vi "My_RIGOL.vi"() -> ()   [LabVIEW 2012]
uses:
  RIGOL DG4000 Series.lvlib
panel:
  out "String 4":string
  out "String 3":string
  out "String 2":string
  out "String":string
  in  "Количество точек":dbl
  in  "Время между импульсами, с":dbl
  in  "Ширина импульса, с":dbl=1000.0
  out "Выход на канал 2":string
  out "Выход на канал 1":string
  in  "Amplitude Unit (0: Vpp) 2":i32(ring) items=["Vpp", "Vrms", "dBm"]
  in  "Amplitude (5 Vpp) 2":dbl=5.0
  in  "Amplitude Unit (0: Vpp)":i32(ring) items=["Vpp", "Vrms", "dBm"]
  in  "Amplitude (5 Vpp)":dbl=5.0
  in  "Частота (1000 Hz)":dbl=1000.0
  in  "VISA resource name":refnum<visa-resource-name>
  # "Chanel 2"
  # "Chanel 1"
  # "ДИОД"
  # "ДЕТЕКТОР"
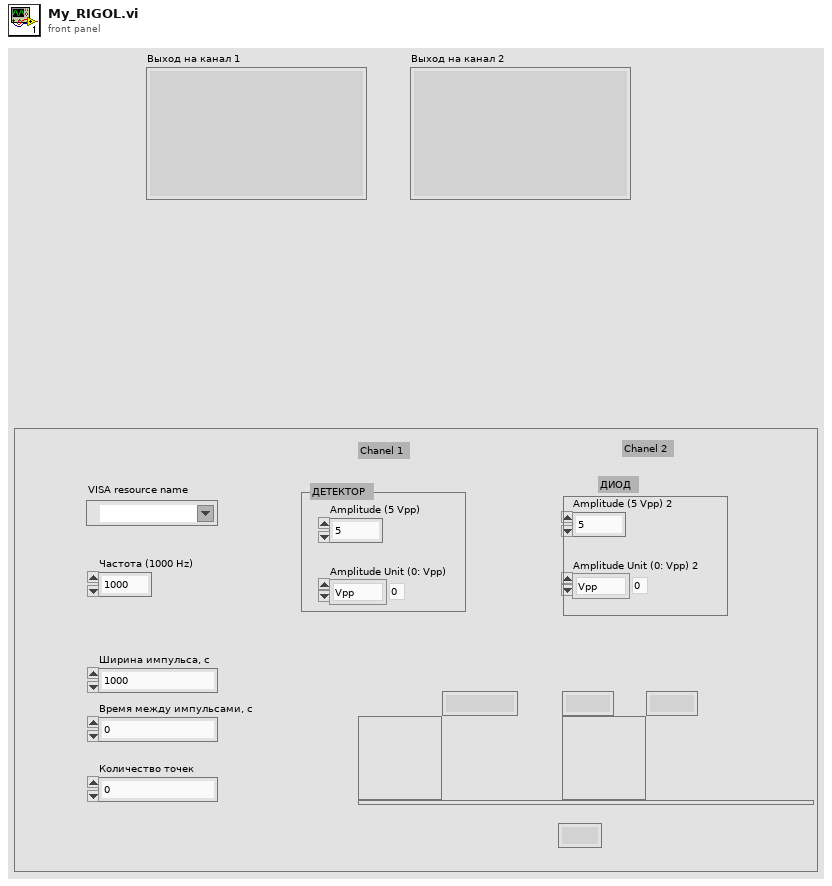
[diagram p1: front panel]
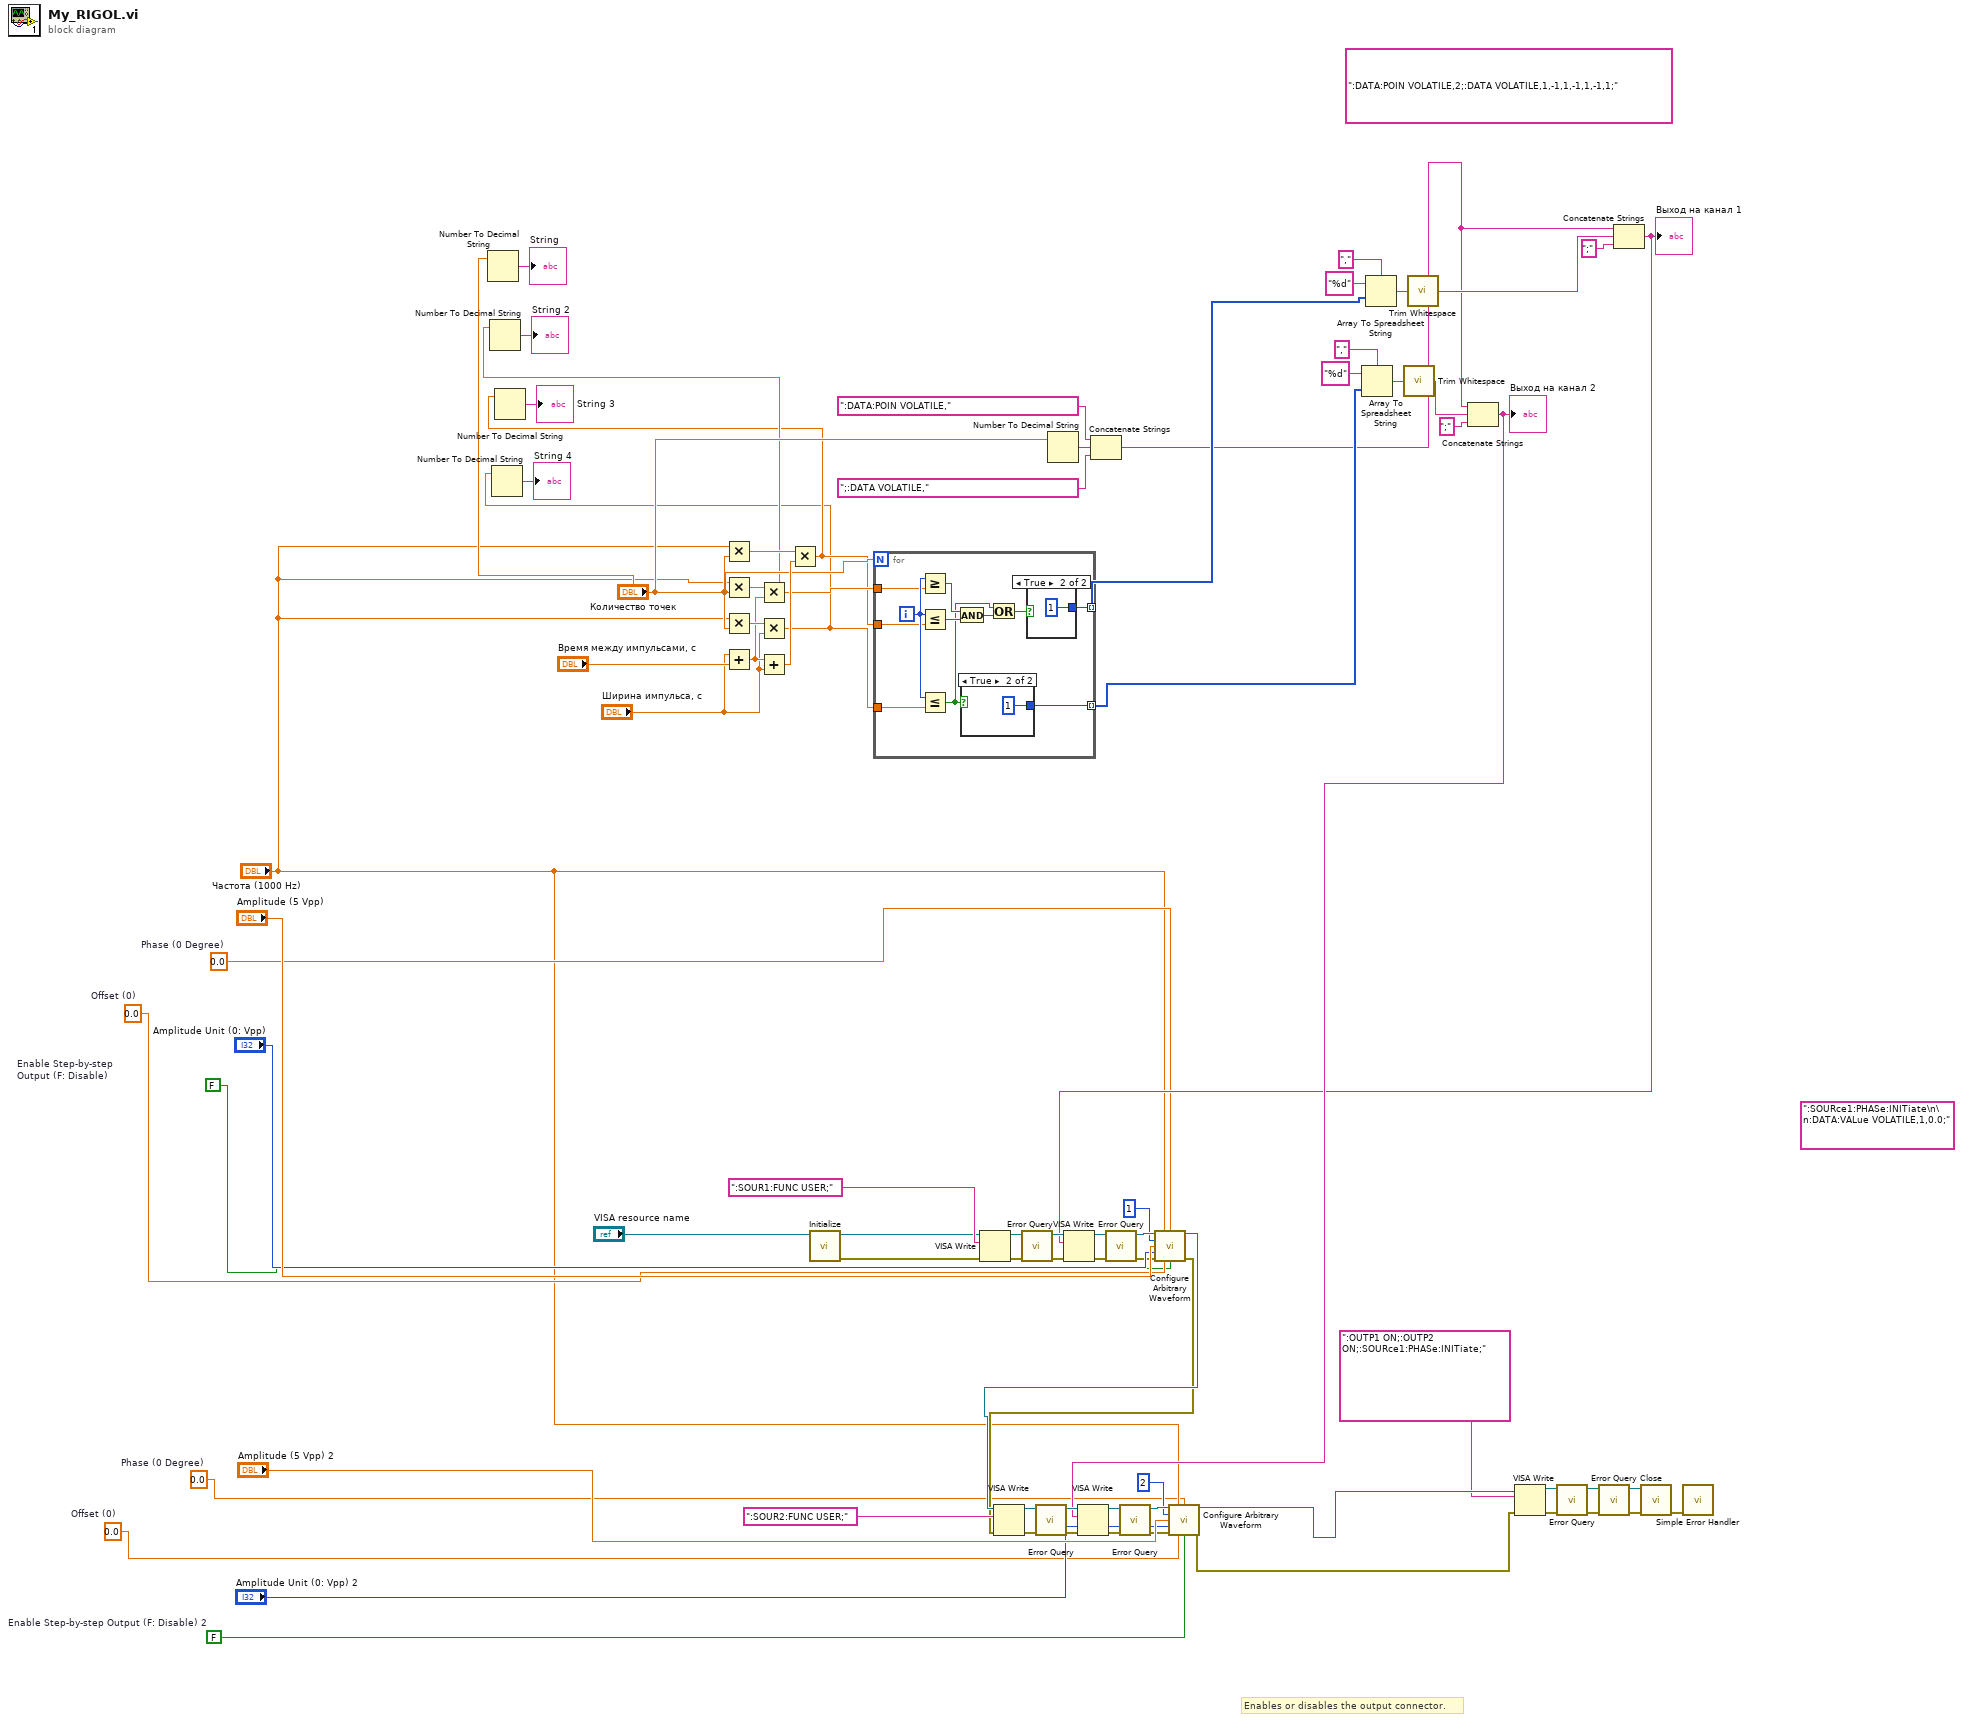
[diagram p0: block diagram]
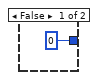
[diagram p2: hidden frame]
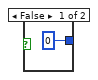
[diagram p3: hidden frame]
diagram:
  w1 = FALSE  # Enable Step-by-step Output (F: Disable) 2
  w2 = FALSE  # Enable Step-by-step Output (F: Disable)
  w3 = 0.0  # Offset (0)
  w4 = 0.0  # Phase (0 Degree)
  w6 = 0.0  # Offset (0)
  w7 = 0.0  # Phase (0 Degree)
  (unwired) ":SOURce1:PHASe:INITiate\n\n:DATA:VALue VOLATILE,1,0.0;"
  (unwired) ":DATA:POIN VOLATILE,2;:DATA VOLATILE,1,-1,1,-1,1,-1,1;"
  # "Enables or disables the output connector."
  n1 = Number To Decimal String(number="Количество точек") -> (decimal integer string=→"String":string)  [unwired: 1 in]
  n2 = Multiply(x="Частота (1000 Hz)", y="Количество точек") -> (x*y=w17:dbl)
  n3 = Multiply(x="Частота (1000 Hz)", y="Количество точек") -> (x*y=w21:dbl)
  n4 = Multiply(x="Частота (1000 Hz)", y="Количество точек") -> (x*y=w22:dbl)
  n5 = Add(x="Ширина импульса, с", y="Время между импульсами, с") -> (x+y=w19:dbl)
  n6 = Multiply(x=w21, y=w19) -> (x*y=w10:dbl)
  n7 = Number To Decimal String(number=w10) -> (decimal integer string=→"String 2":string)  [unwired: 1 in]
  n8 = Multiply(x=w22, y="Ширина импульса, с") -> (x*y=w8:dbl)
  n9 = Number To Decimal String(number=w8) -> (decimal integer string=→"String 4":string)  [unwired: 1 in]
  n10 = Add(x=w19, y="Ширина импульса, с") -> (x+y=w16:dbl)
  n11 = Multiply(x=w17, y=w16) -> (x*y=w9:dbl)
  n12 = Number To Decimal String(number=w9) -> (decimal integer string=→"String 3":string)  [unwired: 1 in]
  n13 = call "Initialize.vi"("VISA resource name"="VISA resource name") -> ("error out"=w50:errorcluster, "VISA resource name out"=w51:refnum<visa-resource-name>)  [unwired: 4 in, 5 out]
  n14 = for {
    N: "Количество точек" -> [_]
    tunnel: [w90] -> w38 mode=indexing
    tunnel: w8 -> [w89]
    tunnel: w10 -> [w83]
    tunnel: w9 -> [w82]
    tunnel: [w80] -> w31 mode=indexing
    i -> [w84]
    n15 = Greater Or Equal?(x=w84, y=w83) -> (x >= y?=w86:bool)
    n16 = Less Or Equal?(x=w84, y=w82) -> (x <= y?=w85:bool)
    n17 = Less Or Equal?(x=w84, y=w89) -> (x <= y?=w81:bool)
    n18 = And(x=w86, y=w85) -> (x .and. y?=w88:bool)
    n19 = case shown="True" w81 {
      tunnel: [0 1] -> w80
      frame False {
      }
      frame True {
      }
    }
    n20 = Or(x=w81, y=w88) -> (x .or. y?=w87:bool)
    n21 = case shown="True" w87 {
      tunnel: [0 1] -> w90
      frame False {
      }
      frame True {
      }
    }
  }
  n22 = VISA Write(VISA resource name=w51, write buffer=":SOUR1:FUNC USER;", error in (no error)=w50) -> (VISA resource name out=w75:refnum<visa-resource-name>, error out=w73:errorcluster)  [unwired: 1 out]
  n23 = call "Error Query.vi"("error in (no error)"=w73, "VISA resource name"=w75) -> ("error out"=w67:errorcluster, "VISA resource name out"=w70:refnum<visa-resource-name>)  [unwired: 8 out]
  n24 = Number To Decimal String(number="Количество точек") -> (decimal integer string=w28:string)  [unwired: 1 in]
  n25 = Concatenate Strings(":DATA:POIN VOLATILE,", w28, ";:DATA VOLATILE,") -> (w25:string)
  n26 = Array To Spreadsheet String(delimiter (Tab)=",", array=w31, 3:"%d") -> (spreadsheet string=w33:string)
  n27 = Array To Spreadsheet String(delimiter (Tab)=",", array=w38, 3:"%d") -> (spreadsheet string=w39:string)
  n28 = call <vilib>:"Trim Whitespace.vi"("string"=w33) -> ("trimmed string"=w32:string)  [unwired: 1 in]
  n29 = call <vilib>:"Trim Whitespace.vi"("string"=w39) -> ("trimmed string"=w37:string)  [unwired: 1 in]
  n30 = Concatenate Strings(w25, w32, ";" ("delimiter (Tab)")) -> (w30:string)
  "Выход на канал 2" <- w30
  n31 = Concatenate Strings(w25, w37, ";" ("delimiter (Tab)")) -> (w29:string)
  "Выход на канал 1" <- w29
  n32 = VISA Write(VISA resource name=w70, write buffer=w29, error in (no error)=w67) -> (VISA resource name out=w69:refnum<visa-resource-name>, error out=w66:errorcluster)  [unwired: 1 out]
  n33 = call "Error Query.vi"("error in (no error)"=w66, "VISA resource name"=w69) -> ("error out"=w65:errorcluster, "VISA resource name out"=w68:refnum<visa-resource-name>)  [unwired: 8 out]
  n34 = call "Configure Arbitrary Waveform.vi"("VISA resource name"=w68, "Frequency (1000 Hz)"="Частота (1000 Hz)", "Phase (0 Degree)"=w7, "Output Channel (1: Channel 1)"=1, "Amplitude (5 Vpp)"="Amplitude (5 Vpp)", "Amplitude Unit (0: Vpp)"="Amplitude Unit (0: Vpp)", "error in (no error)"=w65, "Offset (0)"=w6, "Enable Step-by-step Output (F: Disable)"=w2) -> ("VISA resource name out"=w53:refnum<visa-resource-name>, "error out"=w52:errorcluster)  [unwired: 5 in]
  n35 = VISA Write(VISA resource name=w53, write buffer=":SOUR2:FUNC USER;", error in (no error)=w52) -> (VISA resource name out=w64:refnum<visa-resource-name>, error out=w62:errorcluster)  [unwired: 1 out]
  n36 = call "Error Query.vi"("error in (no error)"=w62, "VISA resource name"=w64) -> ("error out"=w56:errorcluster, "VISA resource name out"=w59:refnum<visa-resource-name>)  [unwired: 8 out]
  n37 = VISA Write(VISA resource name=w59, write buffer=w30, error in (no error)=w56) -> (VISA resource name out=w58:refnum<visa-resource-name>, error out=w55:errorcluster)  [unwired: 1 out]
  n38 = call "Error Query.vi"("error in (no error)"=w55, "VISA resource name"=w58) -> ("error out"=w54:errorcluster, "VISA resource name out"=w57:refnum<visa-resource-name>)  [unwired: 8 out]
  n39 = call "Configure Arbitrary Waveform.vi"("VISA resource name"=w57, "Frequency (1000 Hz)"="Частота (1000 Hz)", "Phase (0 Degree)"=w4, "Output Channel (1: Channel 1)"=2, "Amplitude (5 Vpp)"="Amplitude (5 Vpp) 2", "Amplitude Unit (0: Vpp)"="Amplitude Unit (0: Vpp) 2", "error in (no error)"=w54, "Offset (0)"=w3, "Enable Step-by-step Output (F: Disable)"=w1) -> ("VISA resource name out"=w45:refnum<visa-resource-name>, "error out"=w44:errorcluster)  [unwired: 5 in]
  n40 = VISA Write(VISA resource name=w45, write buffer=":OUTP1 ON;:OUTP2 ON;:SOURce1:PHASe:INITiate;", error in (no error)=w44) -> (VISA resource name out=w47:refnum<visa-resource-name>, error out=w46:errorcluster)  [unwired: 1 out]
  n41 = call "Error Query.vi"("error in (no error)"=w46, "VISA resource name"=w47) -> ("error out"=w24:errorcluster, "VISA resource name out"=w23:refnum<visa-resource-name>)  [unwired: 8 out]
  n42 = call "Error Query.vi"("error in (no error)"=w24, "VISA resource name"=w23) -> ("error out"=w77:errorcluster, "VISA resource name out"=w78:refnum<visa-resource-name>)  [unwired: 8 out]
  n43 = call "Close.vi"("error in (no error)"=w77, "VISA resource name"=w78) -> ("error out"=w76:errorcluster)  [unwired: 9 out]
  n44 = call <vilib>:"Simple Error Handler.vi"("error in (no error)"=w76) -> ()  [unwired: 1 in, 8 out]
